vi "站点信息配置.vi"() -> ()   [LabVIEW 2016]
uses:
  <vilib>/Utility/config.llb/NI_LVConfig.lvlib
panel:
  in  "确定":bool
  in  "纬度：":dbl
  in  "经度：":dbl
  in  "站点名称":string caption="站点名称："
  # "站点信息配置"
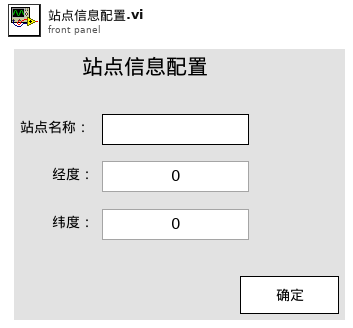
[diagram p1: front panel]
types:
  T1 = typedef "NI_LVConfig.lvlib/Config Data RefNum.ctl" = refnum<k1>
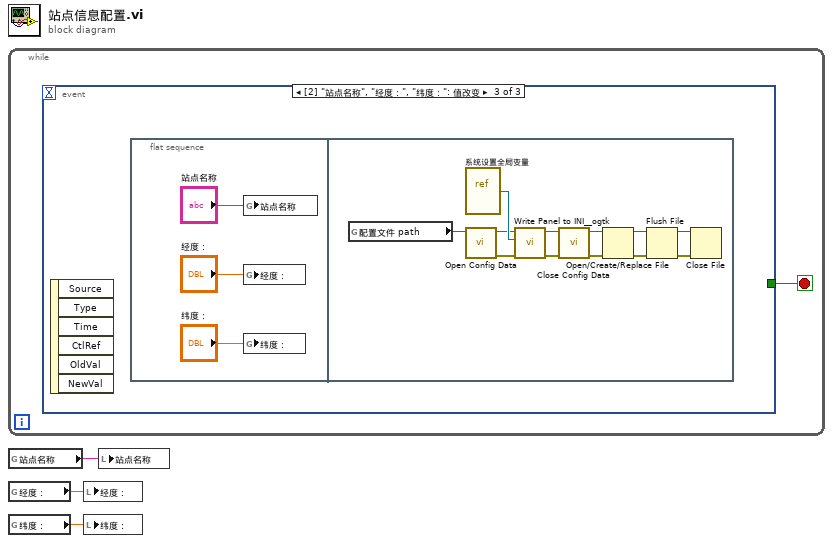
[diagram p0: block diagram]
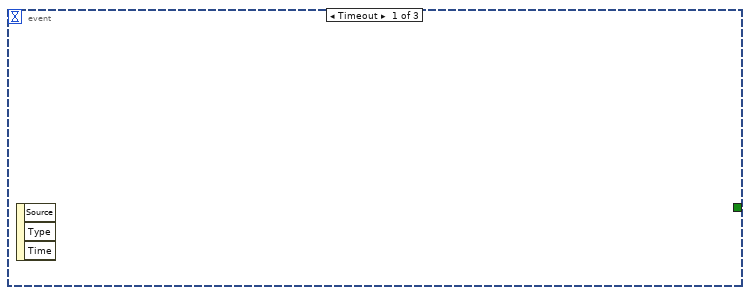
[diagram p2: hidden frame]
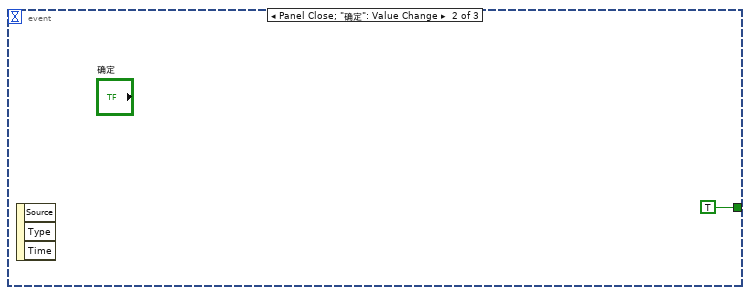
[diagram p3: hidden frame]
diagram:
  n1 = while {
    stop <- w4 stop-if-true
    n2 = event shown="[2] \"站点名称\", \"经度：\", \"纬度：\": 值改变" {
      selector: _ -> [_ _ _]
      dyn-events: _ -> [_ _ _]
      timeout: _ -> [_ _ _]
      tunnel: [_ TRUE _] -> w4
      event Timeout {
        n3 = event-data() -> ()  [unwired: 1 in, 3 out]
      }
      event Panel Close; "确定": Value Change {
        n4 = event-data() -> ()  [unwired: 1 in, 3 out]
      }
      event "站点名称", "经度：", "纬度：": Value Change {
        n5 = event-data() -> ()  [unwired: 1 in, 6 out]
        n6 = flat-sequence {
          frame #0 {
            n7 = global write "系统设置全局变量.vi" "站点名称"("站点名称") -> ()
            n8 = global write "系统设置全局变量.vi" "经度："("经度：") -> ()
            n9 = global write "系统设置全局变量.vi" "纬度："("纬度：") -> ()
          }
          frame #1 {
            n10 = global read "ping全局.vi" "配置文件 path"() -> (w20:path)
            n11 = vi-ref "系统设置全局变量.vi"() -> (w10:refnum<vi>)
            n12 = call <vilib>:"Open Config Data.vi"("configuration file path"=w20) -> ("error out"=w12:errorcluster, "refnum"=w9:T1)  [unwired: 8 in, 1 out]
            n13 = call <userlib>:"Write Panel to INI__ogtk.vi"("error in (no error)"=w12, "VI ref"=w10, "refnum"=w9) -> ("error out"=w13:errorcluster, "refnum out"=w11:T1)  [unwired: 7 in]
            n14 = call <vilib>:"Close Config Data.vi"("error in (no error)"=w13, "refnum"=w11) -> ("error out"=w18:errorcluster, "file path"=w19:path)  [unwired: 8 in]
            n15 = Open/Create/Replace File(file path (use dialog)=w19, error in=w18) -> (refnum out=w15:refnum<file>, error out=w14:errorcluster)  [unwired: 4 in, 1 out]
            n16 = Flush File(refnum=w15, error in=w14) -> (refnum out=w16:refnum<file>, error out=w17:errorcluster)
            n17 = Close File(refnum=w16, error in=w17) -> ()  [unwired: 2 out]
          }
        }
      }
    }
  }
  n18 = global read "系统设置全局变量.vi" "站点名称"() -> (w3:string)
  n19 = global read "系统设置全局变量.vi" "经度："() -> (w1:dbl)
  n20 = global read "系统设置全局变量.vi" "纬度："() -> (w2:dbl)
  n21 = local write "经度："(w1) -> ()
  n22 = local write "纬度："(w2) -> ()
  n23 = local write "站点名称"(w3) -> ()
